vi "FTWLib-nanomsg-Win32.vi"(11 "error in":errorcluster) -> (4 "Integer Size":i32, 15 "error out":errorcluster)   [LabVIEW 2012]
uses:
  ftw-nanomsg/builds/Debug/FTWLib-nanomsg32.dll
panel:
  # "Inputs"
  # "Outputs"
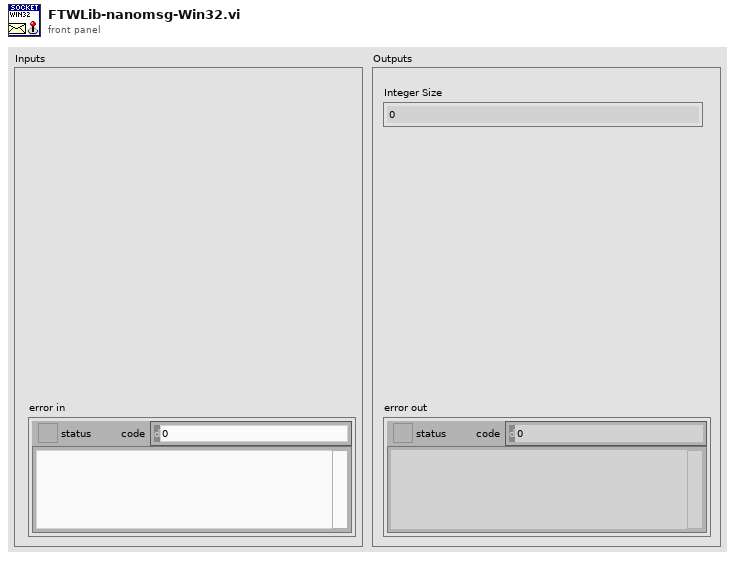
[diagram p1: front panel]
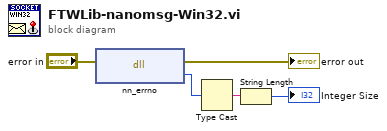
[diagram p0: block diagram]
diagram:
  n1 = dll-call lib="C:/Users/Jack/repo/ftw-nanomsg/builds/Debug/FTWLib-nanomsg32.dll" fn="nn_errno"(error in="error in") -> (error out=→"error out":errorcluster, "Error Code"=w3:i64)  [unwired: 2 in, 1 out]
  n2 = Type Cast(x=w3) -> (*(type *) &x=w2:string)  [unwired: 1 in]
  n3 = String Length(string=w2) -> (length=→"Integer Size":i32)
